vi "H1_Density_Test_V1.vi"() -> ()   [LabVIEW 2020]
uses:
  <instrlib>/niFgen/niFgen.llb/niFgen Output Mode.ctl
  <instrlib>/niFgen/niFgen.llb/niFgen Waveform Type.ctl
  <instrlib>/niFgen/niFgen.llb/niFgen_ctl Trigger DigEdge - Edge Values (Ring).ctl
  <instrlib>/niFgen/niFgen.llb/niFgen_ctl Trigger Source Values (Ring).ctl
  <instrlib>/niFgen/niFgen.llb/niFgen Trigger Mode.ctl
  <instrlib>/niScope/Controls/niScope acquisition type.ctl
  <instrlib>/niScope/Controls/niScope trigger slope.ctl
  <instrlib>/niScope/Controls/niScope trigger source.ctl
  <vilib>/Utility/file.llb/Read Delimited Spreadsheet (DBL).vi
  <instrlib>/niFgen/niFgen.llb/niFgen Create Waveform (DBL).vi
  <instrlib>/niScope/Configure/Trigger/niScope Configure Trigger Edge.vi
  <instrlib>/niFgen/niFgen.llb/niFgen Configure Digital Edge Start Trigger.vi
  <instrlib>/niScope/Acquire/Fetch/niScope Fetch Cluster.vi
panel:
  out "Averaged Pulse Echo":waveform(dbl)(graph)={"t0"=timestamp(0 s since 1904-01-01), "dt"=3.3333333333333333e-06, "Y"=array[1500 elements]} caption="Waveform Graph"
  out "Frequency List (MHz)":dbl[](array[numeric])=[27.46, 27.459, 27.458, 27.457, 27.456, 27.455, 27.454, 27.453, 27.452, 27.451]
  out "Peak Amplitude":dbl[](array[numeric])=[0.7524058042652836, 0.7769028692719315, 0.7777042520634104, 0.7792644046349221, 0.7690737664721656, 0.7587155897528056, 0.7656206143622847, 0.7369389598529605, 0.7186154349892504, 0.700809095893297]
  in  "Pulse Train File":path=path "D:/Single 90 & 180 Degree Pulse Echo.txt"
  in  "Starting Frequency":dbl=27465000.0 caption="Frequency" format="%.4p"
  out "Scan Number":i32=2
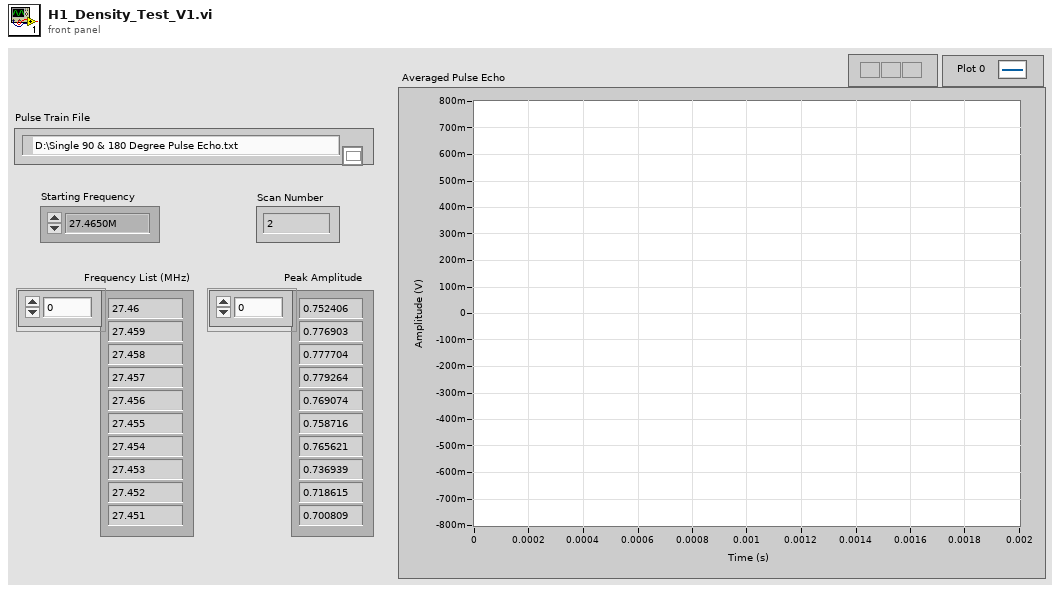
[diagram p1: front panel]
types:
  T1 = typedef "niFgen Output Mode.ctl" = u32
  T2 = typedef "niScope trigger source.ctl" = string
  T3 = typedef "niFgen_ctl Trigger Source Values (Ring).ctl" = string
  T4 = typedef "niScope trigger slope.ctl" = i32
  T5 = typedef "niScope acquisition type.ctl" = i32
  T6 = typedef "niFgen Trigger Mode.ctl" = i32
  T7 = typedef "niFgen_ctl Trigger DigEdge - Edge Values (Ring).ctl" = i32
  T8 = typedef "niFgen Waveform Type.ctl" = i32
  T9 = cluster{"relativeInitialX":dbl, "xIncrement":dbl, "wfm":dbl[]}
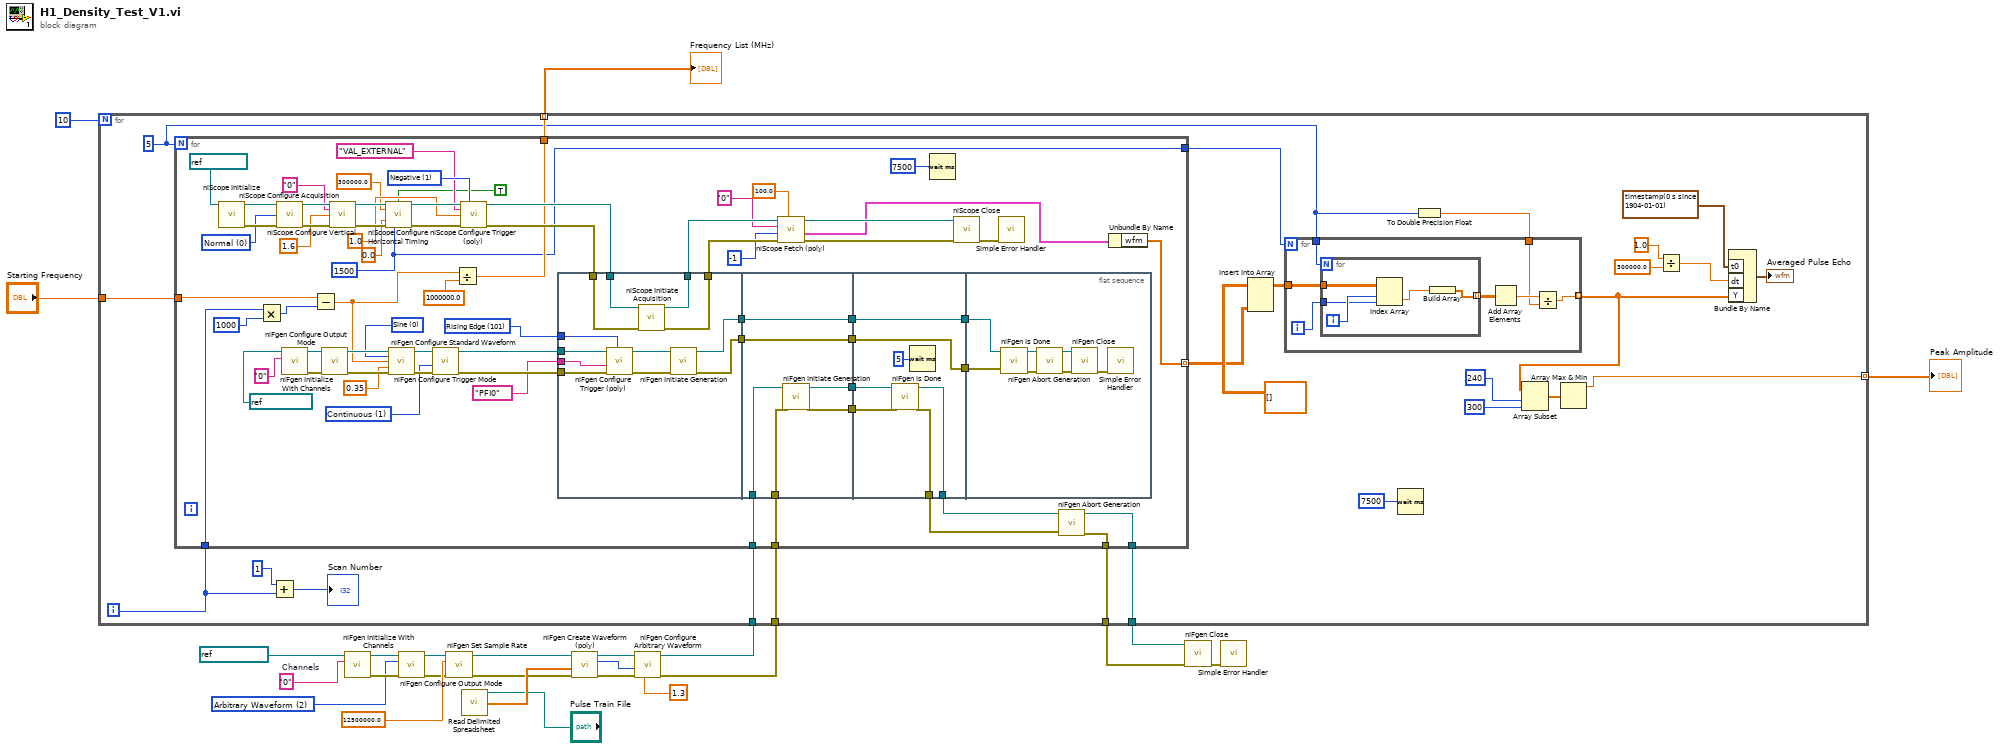
[diagram p0: block diagram]
diagram:
  w11 = "0"  # Channels
  w10 = T1 2 items=["Standard Function", "Frequency List", "Arbitrary Waveform", "Arbitrary Sequence", "Script"] ("output mode")
  n1 = call <instrlib>:"niFgen Initialize With Channels.vi"("Channel Name"=w11, "Resource Name"=refnum<k15> "PulseTrain" ("FGEN Resource Name 2")) -> ("error out"=w14:errorcluster, "Instrument Handle Out"=w15:refnum<k15>)  [unwired: 8 in]
  n2 = call <instrlib>:"niFgen Configure Output Mode.vi"("error in (no error)"=w14, "Output Mode (default: 0=Standard Function)"=w10, "Instrument Handle"=w15) -> ("error out"=w18:errorcluster, "Instrument Handle Out"=w17:refnum<k15>)  [unwired: 6 in]
  n3 = call <instrlib>:"niFgen Set Sample Rate.vi"("error in (no error)"=w18, "Sample Rate (Samp/s)"=12500000.0 ("Sample Rate"), "Instrument Handle"=w17) -> ("error out"=w21:errorcluster, "Instrument Handle Out"=w20:refnum<k15>)  [unwired: 7 in]
  n4 = call-poly <vilib>:"Read Delimited Spreadsheet.vi"("file path (dialog if empty)"="Pulse Train File") -> ("first row"=w22:dbl[])  [unwired: 9 in, 5 out]
  n5 = call-poly <instrlib>:"niFgen Create Waveform (poly).vi"("error in (no error)"=w21, "Waveform Data Array"=w22, "Instrument Handle"=w20) -> ("error out"=w24:errorcluster, "Waveform Handle"=w25:i32, "Instrument Handle Out"=w23:refnum<k15>)  [unwired: 6 in]
  n6 = call <instrlib>:"niFgen Configure Arbitrary Waveform.vi"("Gain"=1.3, "error in (no error)"=w24, "Waveform Handle"=w25, "Instrument Handle"=w23) -> ("error out"=w2:errorcluster, "Instrument Handle Out"=w3:refnum<k15>)  [unwired: 6 in]
  n7 = for {
    N: 10 -> [_]
    tunnel: [w34] -> w8 mode=indexing
    tunnel: "Starting Frequency" -> [w51]
    tunnel: [w50] -> w6 mode=indexing
    tunnel: [w49] -> w5
    tunnel: [w48] -> w4
    tunnel: w3 -> [w47]
    tunnel: w2 -> [w46]
    i -> [w43]
    w31 = 5 ("Number of Scans")
    n8 = for {
      N: w31 -> [_]
      tunnel: w46 -> [w114]
      tunnel: w47 -> [w113]
      tunnel: [w112] -> w49
      tunnel: [w111] -> w48
      tunnel: w51 -> [w73]
      tunnel: [w70] -> w50
      tunnel: w43 -> [w67]
      tunnel: [w66] -> w37 mode=indexing
      tunnel: [w65] -> w36
      w65 = 1500 ("min record length")
      w99 = T4 1 items=["Positive", "Negative"] ("trigger slope")
      w100 = T5 0 items=["Normal"=0, "Flex Res"=1, "DDC"=3] ("acquisition Type")
      w118 = T6 1 items=["Single", "Continuous", "Stepped", "Burst"] ("Trigger Mode (default: 1=continuous)")
      w122 = T7 101 items=["Rising Edge"=101, "Falling Edge"=102] ("Edge (Rising)")
      w123 = T8 0 items=["Sine", "Square", "Triangle", "Ramp Up", "Ramp Down", "DC", "Noise", "User"] ("Waveform")
      n9 = call <instrlib>:"niScope Initialize.vi"("resource name"=refnum<k15> "OScope") -> ("instrument handle"=w101:refnum<k15>, "error out"=w102:errorcluster)  [unwired: 13 in]
      n10 = Multiply(x=w67, y=1000) -> (x*y=w71:i32)
      n11 = call <instrlib>:"niScope Configure Acquisition.vi"("instrument handle"=w101, "acquisition Type"=w100, "error in"=w102) -> ("instrument handle out"=w104:refnum<k15>, "error out"=w105:errorcluster)  [unwired: 11 in]
      n12 = call <instrlib>:"niFgen Initialize With Channels.vi"("Channel Name"="0", "Resource Name"=refnum<k15> "FuncGen" ("Sine Wave Module")) -> ("error out"=w128:errorcluster, "Instrument Handle Out"=w131:refnum<k15>)  [unwired: 8 in]
      n13 = Subtract(x=w73, y=w71) -> (x-y=w69:dbl)
      n14 = call <instrlib>:"niFgen Configure Output Mode.vi"("error in (no error)"=w128, "Instrument Handle"=w131) -> ("error out"=w127:errorcluster, "Instrument Handle Out"=w130:refnum<k15>)  [unwired: 7 in]
      n15 = call <instrlib>:"niScope Configure Vertical.vi"("instrument handle"=w104, "channels"="0", "vertical range"=1.6, "error in"=w105) -> ("instrument handle out"=w106:refnum<k15>, "error out"=w107:errorcluster)  [unwired: 10 in]
      n16 = call <instrlib>:"niScope Configure Horizontal Timing.vi"("instrument handle"=w106, "enforce realtime"=TRUE, "min sample rate"=300000.0, "reference position"=0.0, "error in"=w107, "min record length"=w65) -> ("instrument handle out"=w108:refnum<k15>, "error out"=w109:errorcluster)  [unwired: 8 in]
      n17 = call <instrlib>:"niFgen Configure Standard Waveform.vi"("Instrument Handle"=w130, "Waveform"=w123, "Frequency"=w69, "Amplitude"=0.35, "error in (no error)"=w127) -> ("Instrument Handle Out"=w129:refnum<k15>, "error out"=w126:errorcluster)  [unwired: 9 in]
      n18 = call <instrlib>:"niFgen Configure Trigger Mode.vi"("error in (no error)"=w126, "Trigger Mode (default: 1=continuous)"=w118, "Instrument Handle"=w129) -> ("error out"=w121:errorcluster, "Instrument Handle Out"=w119:refnum<k15>)  [unwired: 7 in]
      n19 = Divide(x=w69, y=1000000.0) -> (x/y=w70:dbl)
      n20 = call-poly <instrlib>:"niScope Configure Trigger (poly).vi"("instrument handle"=w108, "trigger slope"=w99, "trigger source"=T2 "VAL_EXTERNAL", "trigger level"=1.0, "error in"=w109) -> ("instrument handle out"=w93:refnum<k15>, "error out"=w92:errorcluster)  [unwired: 9 in]
      n21 = flat-sequence {
        tunnel: w122 -> [w142]
        tunnel: w121 -> [w141]
        tunnel: T3 "PFI0" ("Source") -> [w140]
        tunnel: w119 -> [w139]
        tunnel: w93 -> [w137]
        tunnel: w92 -> [w136]
        tunnel: [w135] -> w91
        tunnel: [w134] -> w90
        tunnel: [w133] -> w80
        tunnel: [w132] -> w77
        tunnel: w114 -> [w149]
        tunnel: w113 -> [w148]
        tunnel: [w147] -> w84
        tunnel: [w146] -> w83
        tunnel: [w145] -> w81
        tunnel: w80 -> [w145]
        tunnel: [w144] -> w78
        tunnel: w77 -> [w144]
        tunnel: [w155] -> w116
        tunnel: [w154] -> w115
        tunnel: w84 -> [w153]
        tunnel: w83 -> [w152]
        tunnel: [w151] -> w82
        tunnel: w81 -> [w151]
        tunnel: [w150] -> w79
        tunnel: w78 -> [w150]
        tunnel: w82 -> [w158]
        tunnel: w79 -> [w157]
        frame #0 {
          n22 = call-poly <instrlib>:"niFgen Configure Trigger (poly).vi"("Edge (Rising)"=w142, "error in (no error)"=w141, "Source"=w140, "Instrument Handle"=w139) -> ("error out"=w138:errorcluster, "Instrument Handle Out"=w143:refnum<k15>)  [unwired: 6 in]
          n23 = call <instrlib>:"niScope Initiate Acquisition.vi"("instrument handle"=w137, "error in"=w136) -> ("instrument handle out"=w135:refnum<k15>, "error out"=w134:errorcluster)  [unwired: 12 in]
          n24 = call <instrlib>:"niFgen Initiate Generation.vi"("error in (no error)"=w138, "Instrument Handle"=w143) -> ("error out"=w132:errorcluster, "Instrument Handle Out"=w133:refnum<k15>)  [unwired: 8 in]
        }
        frame #1 {
          n25 = call <instrlib>:"niFgen Initiate Generation.vi"("error in (no error)"=w149, "Instrument Handle"=w148) -> ("error out"=w146:errorcluster, "Instrument Handle Out"=w147:refnum<k15>)  [unwired: 8 in]
        }
        frame #2 {
          n26 = call <instrlib>:"niFgen Is Done.vi"("error in (no error)"=w152, "Instrument Handle"=w153) -> ("error out"=w155:errorcluster, "Instrument Handle Out"=w154:refnum<k15>)  [unwired: 7 in, 1 out]
          n27 = Wait (ms)(milliseconds to wait=u32 5) -> ()  [unwired: 1 out]
        }
        frame #3 {
          n28 = call <instrlib>:"niFgen Is Done.vi"("error in (no error)"=w157, "Instrument Handle"=w158) -> ("error out"=w161:errorcluster, "Instrument Handle Out"=w160:refnum<k15>)  [unwired: 7 in, 1 out]
          n29 = call <instrlib>:"niFgen Abort Generation.vi"("error in (no error)"=w161, "Instrument Handle"=w160) -> ("error out"=w162:errorcluster, "Instrument Handle Out"=w163:refnum<k15>)  [unwired: 8 in]
          n30 = call <instrlib>:"niFgen Close.vi"("error in (no error)"=w162, "Instrument Handle"=w163) -> ("error out"=w159:errorcluster)  [unwired: 9 in]
          n31 = call <vilib>:"Simple Error Handler.vi"("error in (no error)"=w159) -> ()  [unwired: 4 in, 5 out]
        }
      }
      n32 = call-poly <instrlib>:"niScope Fetch (poly).vi"("timeout"=100.0, "error in"=w90, "numSamples"=-1, "channels"="0", "instrument handle"=w91) -> ("error out"=w74:errorcluster, "waveform"=w64:T9, "instrument handle out"=w75:refnum<k15>)  [unwired: 3 in, 1 out]
      n33 = Wait (ms)(milliseconds to wait=u32 7500 ("Delay Time (ms)")) -> ()  [unwired: 1 out]
      n34 = call <instrlib>:"niScope Close.vi"("instrument handle"=w75, "error in"=w74) -> ("error out"=w110:errorcluster)  [unwired: 13 in]
      n35 = call <vilib>:"Simple Error Handler.vi"("error in (no error)"=w110) -> ()  [unwired: 4 in, 5 out]
      n36 = call <instrlib>:"niFgen Abort Generation.vi"("error in (no error)"=w116, "Instrument Handle"=w115) -> ("error out"=w112:errorcluster, "Instrument Handle Out"=w111:refnum<k15>)  [unwired: 8 in]
      n37 = Unbundle By Name(w64) -> ("wfm"=w66:dbl[])
    }
    n38 = Add(x=1, y=w43) -> (x+y=→"Scan Number":i32)
    n39 = Insert Into Array(array=dbl[][] [], new element=w37) -> (w39:dbl[][])  [unwired: 2 in]
    n40 = Wait (ms)(milliseconds to wait=u32 7500 ("Delay Time (ms)")) -> ()  [unwired: 1 out]
    n41 = To Double Precision Float(number=w31) -> (double precision float=w35:dbl)
    n42 = for {
      N: w36 -> [_]
      tunnel: w39 -> [w58]
      tunnel: [w54] -> w33 mode=indexing
      tunnel: w31 -> [w53]
      tunnel: w35 -> [w52]
      i -> [w57]
      n43 = for {
        N: w53 -> [_]
        tunnel: w58 -> [w63]
        tunnel: w57 -> [w61]
        tunnel: [w59] -> w56 mode=indexing
        i -> [w62]
        n44 = Index Array(array=w63, index (row)=w62, index (col)=w61) -> (element=w60:dbl)
        n45 = Build Array(w60) -> (w59:dbl[])
      }
      n46 = Add Array Elements(numeric array=w56) -> (sum=w55:dbl)
      n47 = Divide(x=w55, y=w52) -> (x/y=w54:dbl)
    }
    n48 = Array Subset(array=w33, index=240, length=300 ("y")) -> (w42:dbl[])
    n49 = Array Max & Min(array=w42) -> (max value=w34:dbl)  [unwired: 3 out]
    n50 = Divide(x=1.0, y=300000.0) -> (x/y=w30:dbl)
    n51 = Bundle By Name("t0"=timestamp(0 s since 1904-01-01), "dt"=w30, "Y"=w33) -> (→"Averaged Pulse Echo":waveform(dbl))  [unwired: 1 in]
  }
  "Peak Amplitude" <- w8
  "Frequency List (MHz)" <- w6
  n52 = call <instrlib>:"niFgen Close.vi"("error in (no error)"=w5, "Instrument Handle"=w4) -> ("error out"=w9:errorcluster)  [unwired: 9 in]
  n53 = call <vilib>:"Simple Error Handler.vi"("error in (no error)"=w9) -> ()  [unwired: 4 in, 5 out]
